vi "Main.vi"(8 "Error In":errorcluster) -> (0 "Error Out":errorcluster)   [LabVIEW 2018, in "UserInterface.lvlib"]
uses:
  UserInterface.lvlib
  InternalData.ctl
  UserEvents/StopUE.lvlib
  ErrorHandler/ErrorHandler.lvlib
  Controller/Controller.lvlib
panel:
  in  "Tab Control":T1(tab)
  in  "CISCO Stats":string(tree)
  in  "Stop":bool
  in  "Refresh 2":bool
  in  "Configure Mapping":bool
  in  "Report Settings":bool
  in  "Refresh":bool
  in  "Clear Folder":bool
  in  "Cancel Request":bool
  in  "Request Report":bool
  out "Mapped AEs":i32(listbox)
  in  "New AEs":string(combo)
  out "Report Available":bool
  out "Available weeks":string
  out "Request ID":string
  out "Update Required?":bool=TRUE
  in  "Available Reports":i32(listbox)
  in  "Display Stats":bool
  out "Data Display":T2(array[cluster]) {"Open SRs" scale=0.0..40.0; "Solved in more then 5 Workdays" scale=0.0..40.0; "In Work SRs" scale=0.0..40.0; "Solved Within 5 workdays" scale=0.0..40.0; "New SRs" scale=0.0..40.0}
  in  "Year":i16=1 min=1904 max=2019 step=1
  in  "Week":i16=1 min=1 max=52 step=1
  out "Open SRs":u32(colorbox)=16711680
  out "Solved in more then 5 workdays":u32(colorbox)=16753962
  out "In work":u32(colorbox)=9567230
  out "Solved within 5 workdays":u32(colorbox)=6618880
  out "New SRs":u32(colorbox)=16860
  in  "Save to File":bool
  in  "Filters Configuration":bool
  in  "View Selection":T3(ring)
  in  "SRs Queue":string(tree)
  out "End Date":timestamp format="%<%x>T"
  out "Start Date":timestamp format="%<%x>T"
  in  "SR Linkage":string[][](table)
  in  "AE Stats":string[][](table)
  in  "KCS Linkage":bool
  in  "Filters Configuration 2":bool
  in  "AE Selection":enum16{""}(ring)
  in  "SRs View":string(tree)
  in  "DoSomething":bool
  in  "STOP":bool
  out "Reply Data":dbl
  in  "WaitOnReply":bool
  out "OracleReply":i32
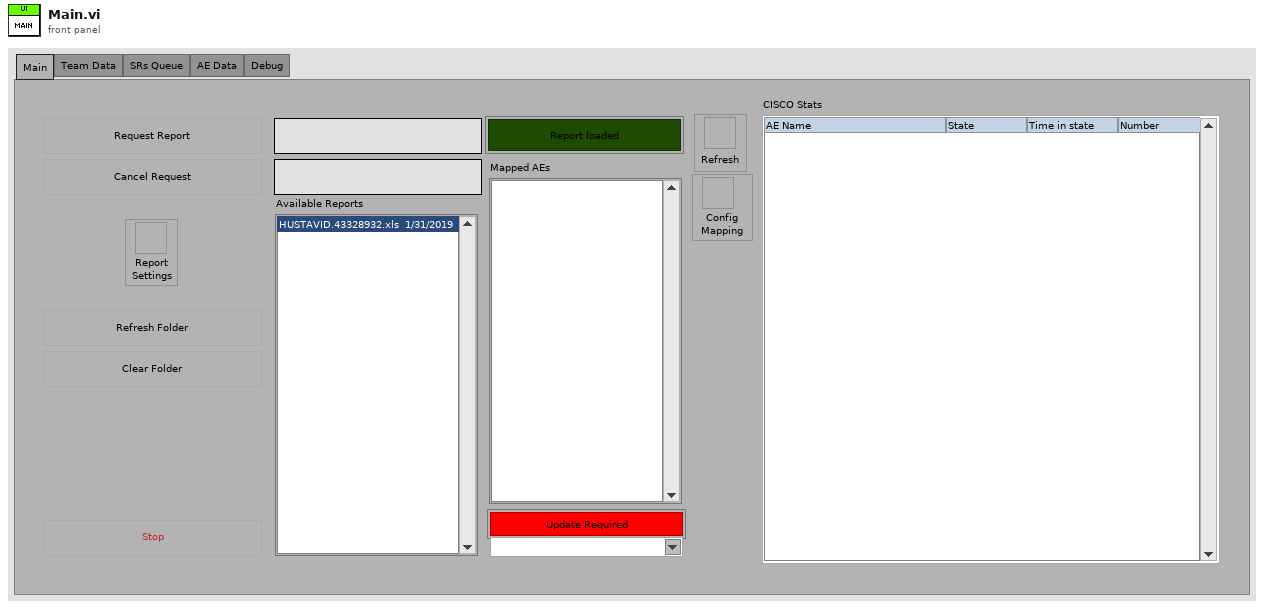
[diagram p1: front panel]
types:
  T1 = enum32{"Main", "Team Data", "SRs Queue", "AE Data", "Debug"}
  T2 = cluster{"New SRs":u8, "Solved Within 5 workdays":u8, "In Work SRs":u8, "Solved in more then 5 Workdays":u8, "Open SRs":u8, "AE-Team":string}[]
  T3 = enum16{"Open", "In Work", "View All", "Neglected"}
  T4 = typedef "UserInterface.lvlib/InternalData.ctl" = cluster{"Status":string}
  T5 = typedef "UserInterface.lvlib/States_Module.ctl" = enum16{"DoSomething", "Shutdown", "Initialize", "RequestOracleReport"}
  T6 = typedef "UserInterface.lvlib/MessageData.ctl" = cluster{"State":T5, "Payload":variant, "WaitOnReply":bool, "ReplyNotif":refnum<notifier>}
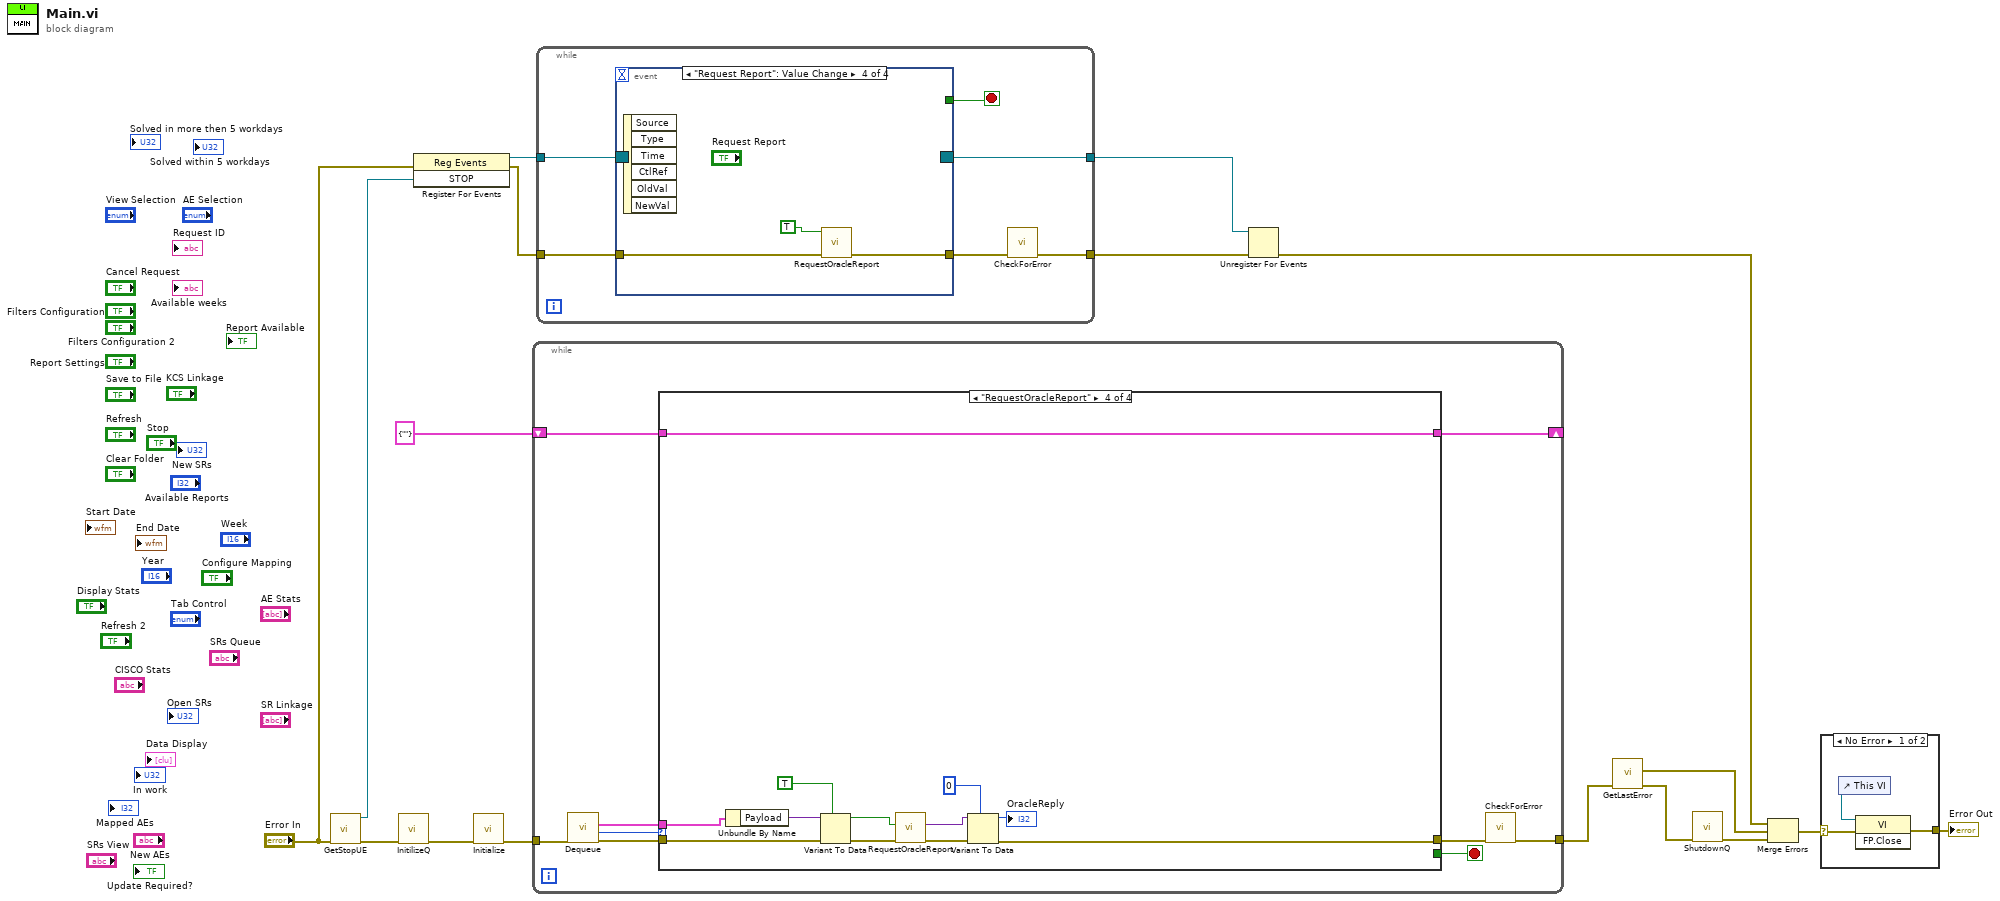
[diagram p0: block diagram]
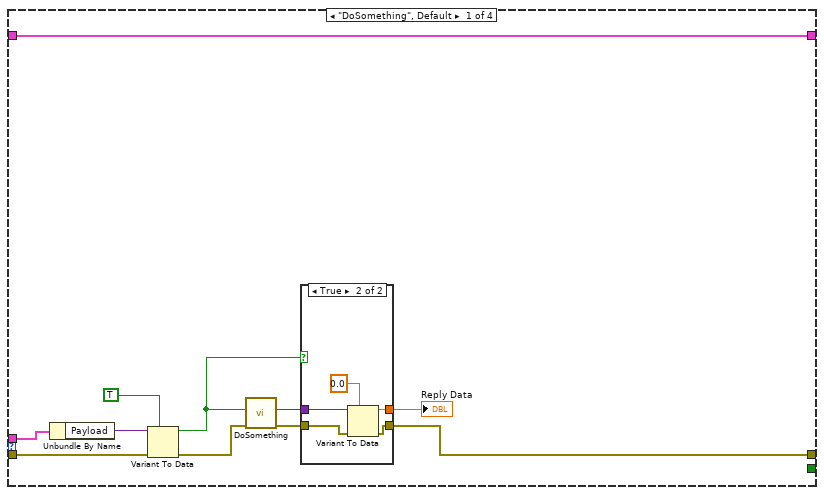
[diagram p3: hidden frame]
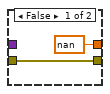
[diagram p4: hidden frame]
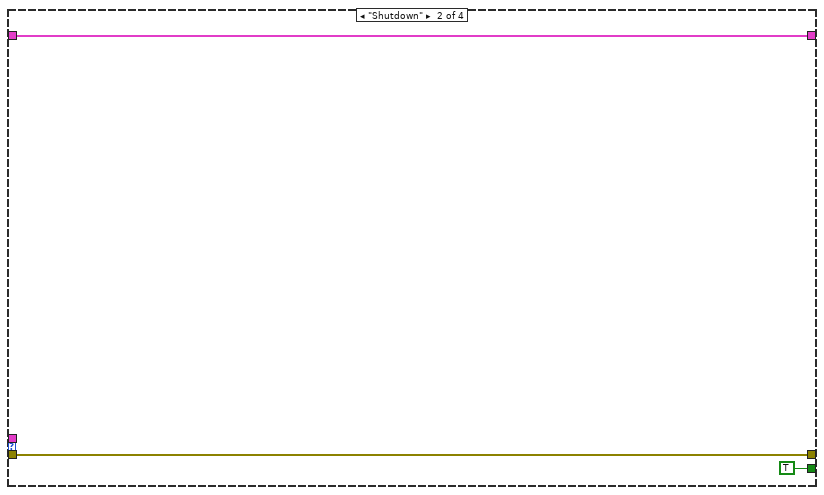
[diagram p5: hidden frame]
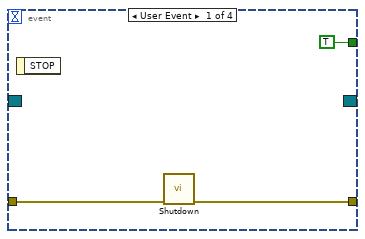
[diagram p7: hidden frame]
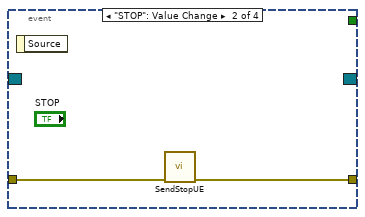
[diagram p8: hidden frame]
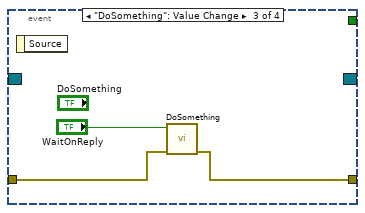
[diagram p9: hidden frame]
diagram:
  n1 = call "GetStopUE.vi"("Error In"="Error In") -> ("Error Out"=w14:errorcluster, "STOP"=w17:refnum<user-event>)  [unwired: 9 in]
  n2 = call "InitilizeQ.vi"("Error In"=w14) -> ("Error Out"=w12:errorcluster)  [unwired: 10 in]
  n3 = register-events(error in="Error In", w17) -> (reference out=w16:refnum<event-registration>, error out=w15:errorcluster)  [unwired: 1 in]
  n4 = call "Initialize.vi"("Error In"=w12) -> ("error out"=w11:errorcluster)  [unwired: 9 in, 1 out]
  n5 = while {
    tunnel: w11 -> [w26]
    tunnel: [w19] -> w8
    shift-right: [w21] -> _
    shift-left: T4 {"Status"=""} ("InternalData") -> [w22]
    stop <- w23 stop-if-true
    n6 = call "Dequeue.vi"("Error In"=w26) -> ("error out"=w25:errorcluster, "State"=w24:T5, "Data out"=w18:T6)  [unwired: 8 in]
    n7 = case shown="\"RequestOracleReport\"" w24 {
      tunnel: w25 -> [w32 w46 w49 w58]
      tunnel: [_ TRUE _ _] -> w23
      tunnel: [w28 w46 w49 w50] -> w20
      tunnel: w22 -> [w37 w45 w48 w61]
      tunnel: [w37 w45 w48 w61] -> w21
      tunnel: w18 -> [w33 _ _ w57]
      frame "DoSomething", Default {
        n8 = Unbundle By Name(w33) -> ("Payload"=w31:variant)
        n9 = Variant To Data(error in=w32, type=TRUE, Variant=w31) -> (data=w27:bool, error out=w29:errorcluster)
        n10 = call "DoSomething.vi"("Error In"=w29, "WaitOnReply"=w27) -> ("error out"=w36:errorcluster, "Reply"=w35:variant)  [unwired: 8 in]
        n11 = case shown="True" w27 {
          tunnel: w36 -> [w39 w43]
          tunnel: w35 -> [_ w44]
          tunnel: [w39 w41] -> w28
          tunnel: [nan ("Reply Data") w40] -> w34
          frame False {
          }
          frame True {
            n12 = Variant To Data(error in=w43, type=0.0 ("Reply Data"), Variant=w44) -> (data=w40:dbl, error out=w41:errorcluster)
          }
        }
        "Reply Data" <- w34
      }
      frame "Shutdown" {
      }
      frame "Initialize" {
      }
      frame "RequestOracleReport" {
        n13 = Unbundle By Name(w57) -> ("Payload"=w60:variant)
        n14 = Variant To Data(error in=w58, type=TRUE, Variant=w60) -> (data=w55:bool, error out=w56:errorcluster)
        n15 = call "RequestOracleReport.vi"("Error In"=w56, "WaitOnReply"=w55) -> ("error out"=w51:errorcluster, "Reply"=w54:variant)  [unwired: 8 in]
        n16 = Variant To Data(error in=w51, type=0, Variant=w54) -> (data=→"OracleReply":i32, error out=w50:errorcluster)
      }
    }
    n17 = call "CheckForError.vi"("Error In"=w20) -> ("error out"=w19:errorcluster)  [unwired: 10 in]
  }
  n18 = while {
    tunnel: w16 -> [w67]
    tunnel: w15 -> [w65]
    tunnel: [w62] -> w10
    tunnel: [w64] -> w9
    stop <- w66 stop-if-true
    n19 = event shown="[3] \"Request Report\": Value Change" {
      selector: w67 -> [_ _ _ _]
      dyn-events: [_ _ _ _] -> w64
      timeout: _ -> [_ _ _ _]
      tunnel: [TRUE _ _ _] -> w66
      tunnel: w65 -> [w69 w72 w75 w78]
      tunnel: [w68 w71 w74 w77] -> w63
      event User Event {
        n20 = event-data() -> ()  [unwired: 1 in, 1 out]
        n21 = call "Shutdown.vi"("Error In"=w69) -> ("error out"=w68:errorcluster)  [unwired: 9 in, 1 out]
      }
      event "STOP": Value Change {
        n22 = event-data() -> ()  [unwired: 1 in, 1 out]
        n23 = call "SendStopUE.vi"("Error In"=w72) -> ("Error Out"=w71:errorcluster)  [unwired: 10 in]
      }
      event "DoSomething": Value Change {
        n24 = event-data() -> ()  [unwired: 1 in, 1 out]
        n25 = call "DoSomething.vi"("Error In"=w75, "Payload"="WaitOnReply") -> ("error out"=w74:errorcluster)  [unwired: 8 in, 1 out]
      }
      event "Request Report": Value Change {
        n26 = event-data() -> ()  [unwired: 1 in, 6 out]
        n27 = call "RequestOracleReport.vi"("Error In"=w78, "Payload"=TRUE) -> ("error out"=w77:errorcluster)  [unwired: 8 in, 1 out]
      }
    }
    n28 = call "CheckForError.vi"("Error In"=w63) -> ("error out"=w62:errorcluster)  [unwired: 10 in]
  }
  n29 = Unregister For Events(event registration refnum=w9, error in=w10) -> (error out=w4:errorcluster)
  n30 = call "GetLastError.vi"("Error In"=w8) -> ("error IO"=w7:errorcluster, "Last Error"=w5:errorcluster)  [unwired: 9 in]
  n31 = call "ShutdownQ.vi"("Error In"=w7) -> ("Error Out"=w6:errorcluster)  [unwired: 10 in]
  n32 = Merge Errors(w4, w5, w6) -> (w1:errorcluster)
  n33 = case shown="No Error" w1 {
    selector: w1 -> [w81 w82]
    tunnel: [w80 w82] -> w2
    frame No Error {
      n34 = control-ref of="This VI"() -> (w79:refnum<vi>)
      n35 = invoke class="VI" method="FP.Close"(reference=w79, error in=w81) -> (error out=w80:errorcluster)  [unwired: 1 in, 2 out]
    }
    frame Error {
    }
  }
  "Error Out" <- w2
